vi "_Open Named Pipe.vi"(8 "error in":errorcluster, 11 "Path":path) -> (0 "error out":errorcluster, 3 "fd out":u64)   [LabVIEW 2020, in "NI_Subprocess.lvlib" / "Subprocess.lvclass"]
uses:
  <vilib>/Subprocess/Subprocess/Subprocess.lvclass
  lviosrg.dll
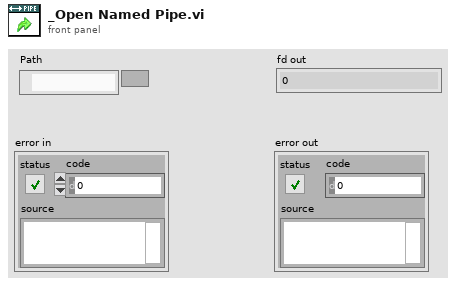
[diagram p1: front panel]
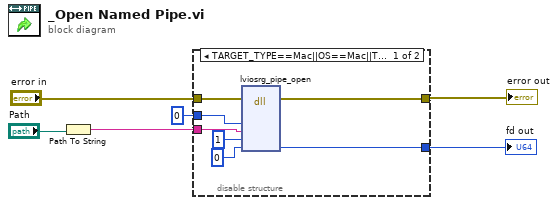
[diagram p0: block diagram]
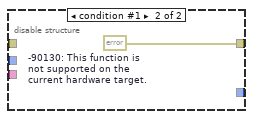
[diagram p2: hidden frame]
diagram:
  n1 = Path To String(path="Path") -> (string=w4:string)
  n2 = disable-structure "Conditional Disable Structure" shown="TARGET_TYPE==Mac||OS==Mac||TARGET_TYPE==Windows||OS==Win||TARGET_TYPE==Unix||OS==Linux" {
    disable-tunnel: [w12 _] -> w3
    disable-tunnel: [w11 w14] -> w2
    disable-tunnel: 0 ("errno") -> [w10 _]
    disable-tunnel: w4 -> [w8 _]
    disable-tunnel: "error in" -> [w7 _]
    frame condition #0 (active) {
      n3 = dll-call lib="lviosrg.*" fn="lviosrg_pipe_open"(error in=w7, "errno"=w10, "path"=w8, "reading"=i8 1, "fd"=u64 0) -> (error out=w11:errorcluster, "fd"=w12:u64)  [unwired: 8 in, 1 out]
    }
    frame condition #1 {
      w14 = errorcluster {"status"=TRUE, "code"=-90130, "source"=""}  # -90130: This function is not supported on the current hardware target.
    }
  }
  "error out" <- w2
  "fd out" <- w3
